vi "queue_loop.vi"() -> ()   [LabVIEW 2014]
uses:
  <vilib>/vision/driver/NI_Vision_Acquisition_Software.lvlib
panel:
  in  "Camera Properties":T1
  in  "stop 2":bool
  out "Image":T2(plugin-control)
  out "calibration time":u32
  in  "stop":bool
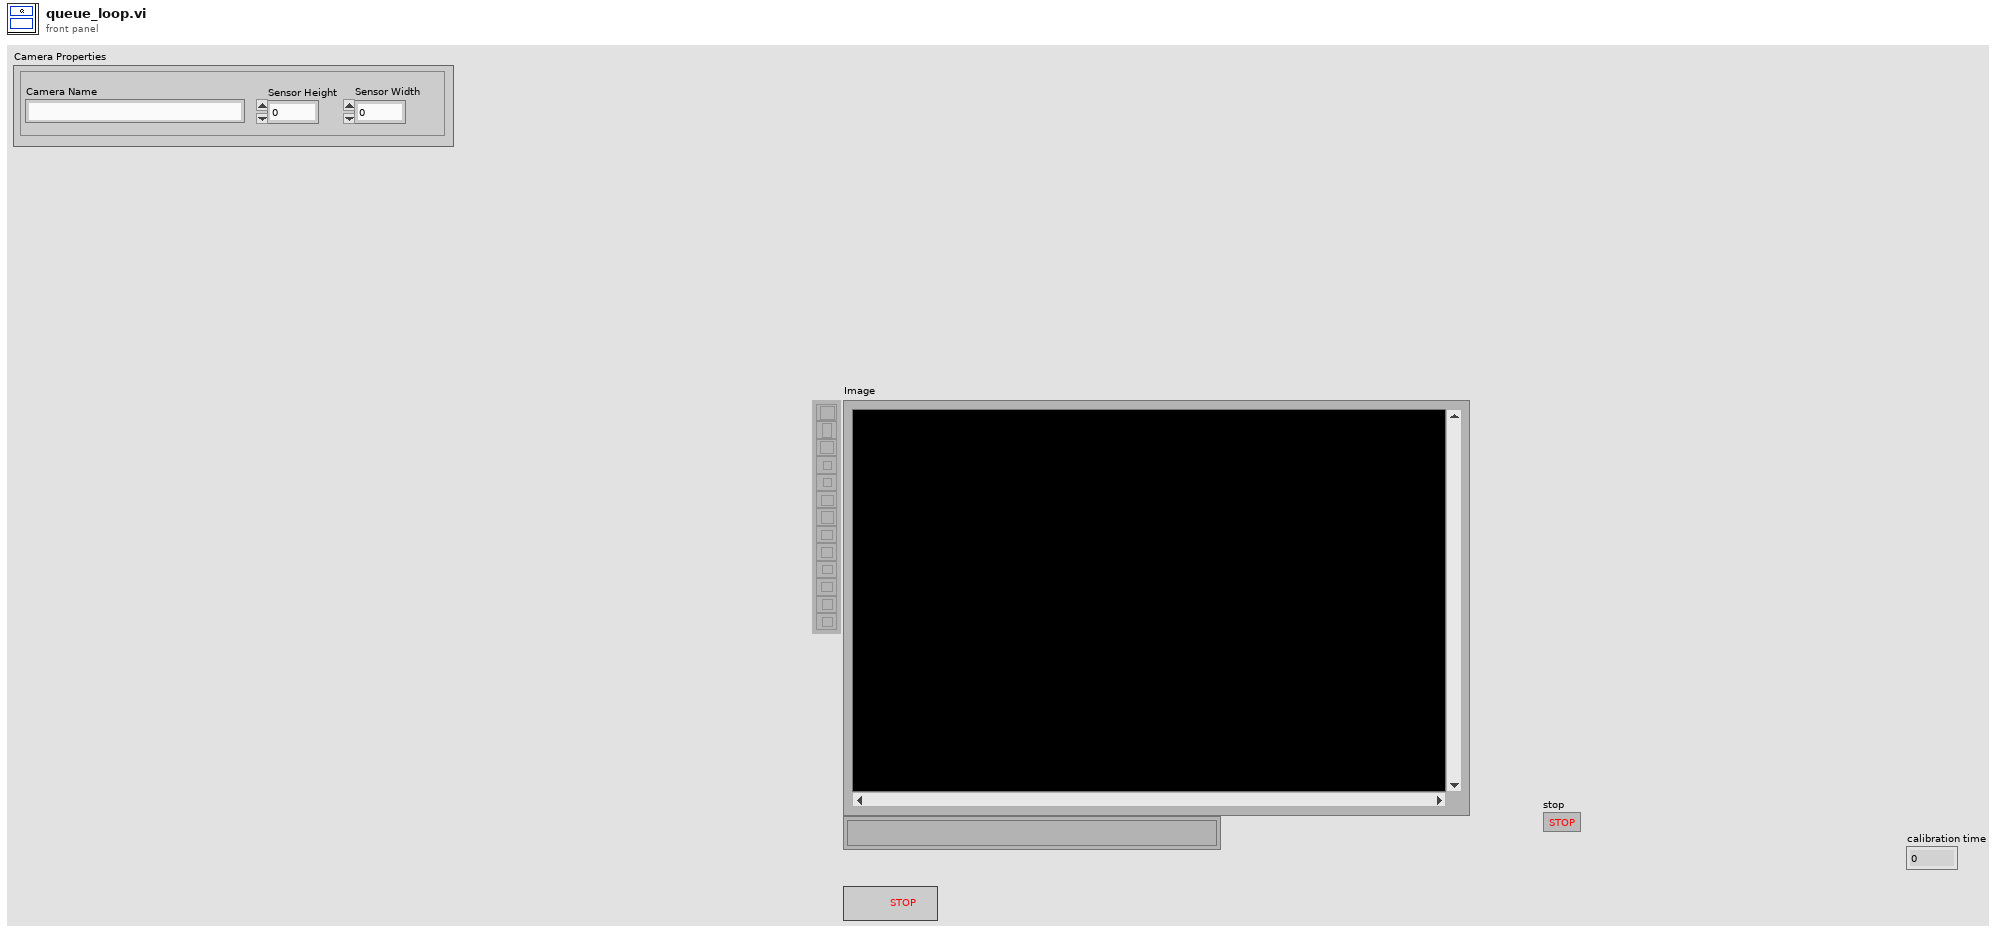
[diagram p1: front panel]
types:
  T1 = cluster{"Camera Name":string, "Sensor Height":u32, "Sensor Width":u32}
  T2 = typedef "IMAQ Image.ctl" = refnum<image>
  T3 = typedef "Image Type" = u32
  T4 = typedef "IMAQdx.ctl" = refnum<k21>
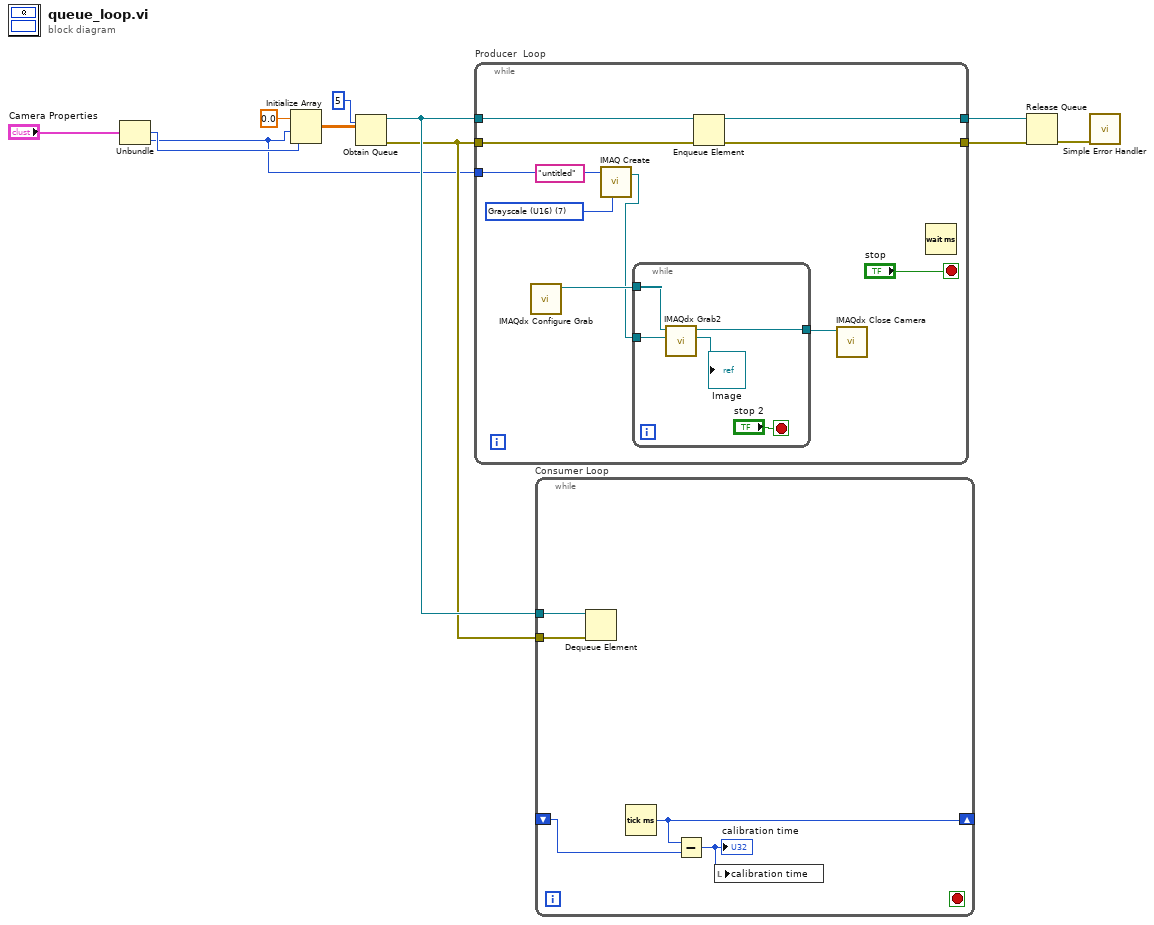
[diagram p0: block diagram]
diagram:
  n1 = Unbundle("Camera Properties") -> ("Sensor Height"=w2:u32, "Sensor Width"=w1:u32)  [unwired: 1 out]
  n2 = Initialize Array(0.0 ("element"), w1, w2) -> (w10:dbl[][])
  n3 = Obtain Queue(max queue size (-1, unlimited)=5, element data type=w10) -> (queue out=w8:refnum<queue>, error out=w7:errorcluster)  [unwired: 3 in, 1 out]
  n4 = while "Producer  Loop" {
    tunnel: w8 -> [w21]
    tunnel: w7 -> [w18]
    tunnel: [w20] -> w6
    tunnel: [w19] -> w5
    tunnel: w1 -> [w17]
    stop <- "stop" stop-if-true
    w15 = T3 7 items=["Grayscale (U8)", "Grayscale (I16)", "Grayscale (SGL)", "Complex (CSG)", "RGB (U32)", "HSL (U32)", "RGB (U64)", "Grayscale (U16)"] ("Image Type")
    # "Pro"
    n5 = call <vilib>:"IMAQdx Configure Grab.vi"() -> ("Session Out"=w13:T4)  [unwired: 10 in, 1 out]
    n6 = call "IMAQ Create"("Border Size"=w17, "Image Name"="untitled", "Image Type"=w15) -> ("New Image"=w12:T2)  [unwired: 2 in, 1 out]
    n7 = while {
      tunnel: w13 -> [w26]
      tunnel: [w25] -> w14
      tunnel: w12 -> [w23]
      stop <- "stop 2" stop-if-true
      n8 = call <vilib>:"IMAQdx Grab2.vi"("Image In"=w23, "Session In"=w26) -> ("Image Out"=→"Image":T2, "Session Out"=w25:T4)  [unwired: 6 in, 2 out]
    }
    n9 = Enqueue Element(queue=w21, error in (no error)=w18) -> (queue out=w20:refnum<queue>, error out=w19:errorcluster)  [unwired: 2 in, 1 out]
    n10 = call <vilib>:"IMAQdx Close Camera.vi"("Session In"=w14) -> ()  [unwired: 10 in, 1 out]
    n11 = Wait (ms)() -> ()  [unwired: 1 in, 1 out]
  }
  n12 = while "Consumer Loop" {
    tunnel: w8 -> [w32]
    tunnel: w7 -> [w31]
    shift-right: [w29] -> _
    shift-left: _ -> [w30]
    stop <- _ stop-if-true
    n13 = Dequeue Element(queue=w32, error in (no error)=w31) -> ()  [unwired: 1 in, 4 out]
    n14 = Tick Count (ms)() -> (millisecond timer value=w29:u32)
    n15 = Subtract(x=w29, y=w30) -> (x-y=w28:u32)
    "calibration time" <- w28
    n16 = local write "calibration time"(w28) -> ()
  }
  n17 = Release Queue(queue=w6, error in (no error)=w5) -> (error out=w4:errorcluster)  [unwired: 1 in, 2 out]
  n18 = call <vilib>:"Simple Error Handler.vi"("error in (no error)"=w4) -> ()  [unwired: 4 in, 5 out]
